vi "init_hw.vi"(8 "error in (no error)":errorcluster, 11 "stresing in":refnum<class "stresing.lvclass">) -> (0 "error out":errorcluster, 2 "success ?":bool=TRUE, 3 "stresing out":refnum<class "stresing.lvclass">)   [LabVIEW 2019, in "stresing.lvlib" / "stresing.lvclass"]
uses:
  stresing.lvclass
  stresing.lvclass/stresing.ctl
panel:
  out "wait time":dbl
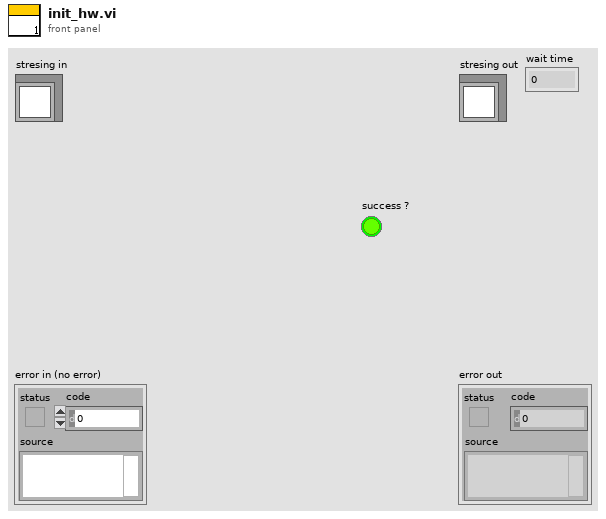
[diagram p1: front panel]
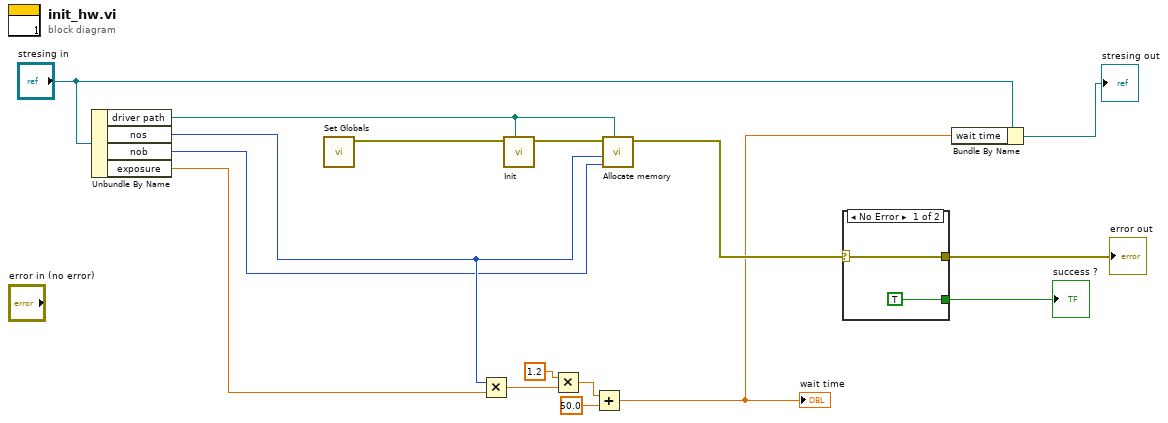
[diagram p0: block diagram]
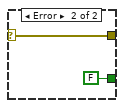
[diagram p2: hidden frame]
diagram:
  n1 = Unbundle By Name("stresing in") -> ("driver path"=w1:path, "nos"=w8:u32, "nob"=w7:u32, "exposure"=w6:dbl)
  n2 = call "Set Globals.vi"() -> ("Camera error out"=w16:errorcluster)  [unwired: 11 in]
  n3 = Multiply(x=w8, y=w6) -> (x*y=w12:dbl)
  n4 = call "Init.vi"("driver path in"=w1, "Camera error in"=w16) -> ("Camera error out"=w15:errorcluster)  [unwired: 9 in]
  n5 = Multiply(x=1.2, y=w12) -> (x*y=w10:dbl)
  n6 = Add(x=w10, y=50.0) -> (x+y=w2:dbl)
  "wait time" <- w2
  n7 = call "Allocate memory.vi"("path in"=w1, "nob"=w7, "nos"=w8, "Camera error in"=w15) -> ("Camera error out"=w14:errorcluster)  [unwired: 7 in]
  n8 = case shown="No Error" w14 {
    selector: w14 -> [w17 w19]
    tunnel: [TRUE FALSE] -> w13
    tunnel: [w17 w19] -> w5
    frame No Error {
    }
    frame Error {
    }
  }
  "error out" <- w5
  "success ?" <- w13
  n9 = Bundle By Name(cluster="stresing in", "wait time"=w2) -> (→"stresing out":refnum<class "stresing.lvclass">)
